vi "PCUI.vi"() -> ()   [LabVIEW 2013, in "PLTarget PC.lvclass"]
doc: "This VI is a template of the minimun components for a node UI.\nIt shows how to use the queue and the user event."
uses:
  PLTarget PC.lvclass
  <vilib>/NI/Configuration Framework/Node/NodeRef.ctl
  <vilib>/NI/Configuration Framework/Node/NISE_CEF_Node.lvclass
  <vilib>/NI/AMC/Message Queue.ctl
  <vilib>/NI/AMC/Message.ctl
  <vilib>/NI/Tools/Keyed Array/KeyedArray.ctl
  <vilib>/NI/Configuration Framework/Node/UserEventRef.ctl
  <vilib>/NI/Configuration Framework/Controls/EventCluster.ctl
  <vilib>/NI/Configuration Framework/Node/RefreshUIEvent.ctl
  <vilib>/NI/Configuration Framework/Node/CacheState.ctl
  <vilib>/NI/Configuration Framework/Node/StopEvent.ctl
  <vilib>/NI/Configuration Framework/Node/NodeChangeEvent.ctl
  <vilib>/Utility/miscctls.llb/LVPositionTypeDef.ctl
  PLTarget PC.lvclass/PLTarget PC.ctl
  Framework Configuration Classes/target configuration/PL_Target Configuration.lvclass/PL_Target Configuration.ctl
  <vilib>/NI/Configuration Framework/serializable node/NISE_CEF_serializable node.lvclass
  <vilib>/NI/Tag Bus Module Framework/root configuration/TBM configuration.lvclass
  <vilib>/NI/Configuration Framework/serializable configuration/set alias.vi
  <vilib>/NI/Configuration Framework/serializable configuration/get alias.vi
  <vilib>/NI/Configuration Framework/serializable configuration/NISE_CEF_serializable configuration.lvclass
  Framework Configuration Classes/target configuration/PL_Target Configuration.lvclass
  <vilib>/NI/DCAF UI Toolkit/Controls/DCAF UI Elements.lvlib
  <vilib>/NI/Tools/Keyed Array/Tools_KeyedArray.lvlib
  <vilib>/NI/AMC/AMC.lvlib
  <vilib>/NI/Configuration Framework/NISE_CEF_TreeControl.lvlib
panel:
  in  "Top Level Tab Control":enum32{"Configuration"}(tab)
  in  "Name":string
  in  "Includes file path":path
  in  "path to deploy on target relative to root (c:\\ or /home/lvuser/)":path
  in  "generate includes file":bool
  in  "node change":T1
  in  "stop event":T2
  in  "cache state":T3
  in  "refresh UI":T4
  in  "open fp?":bool=TRUE
  in  "user event":T5
  in  "main queue":T6
  in  "node ref":T7
  # "Target Information"
  # "Deployment Settings"
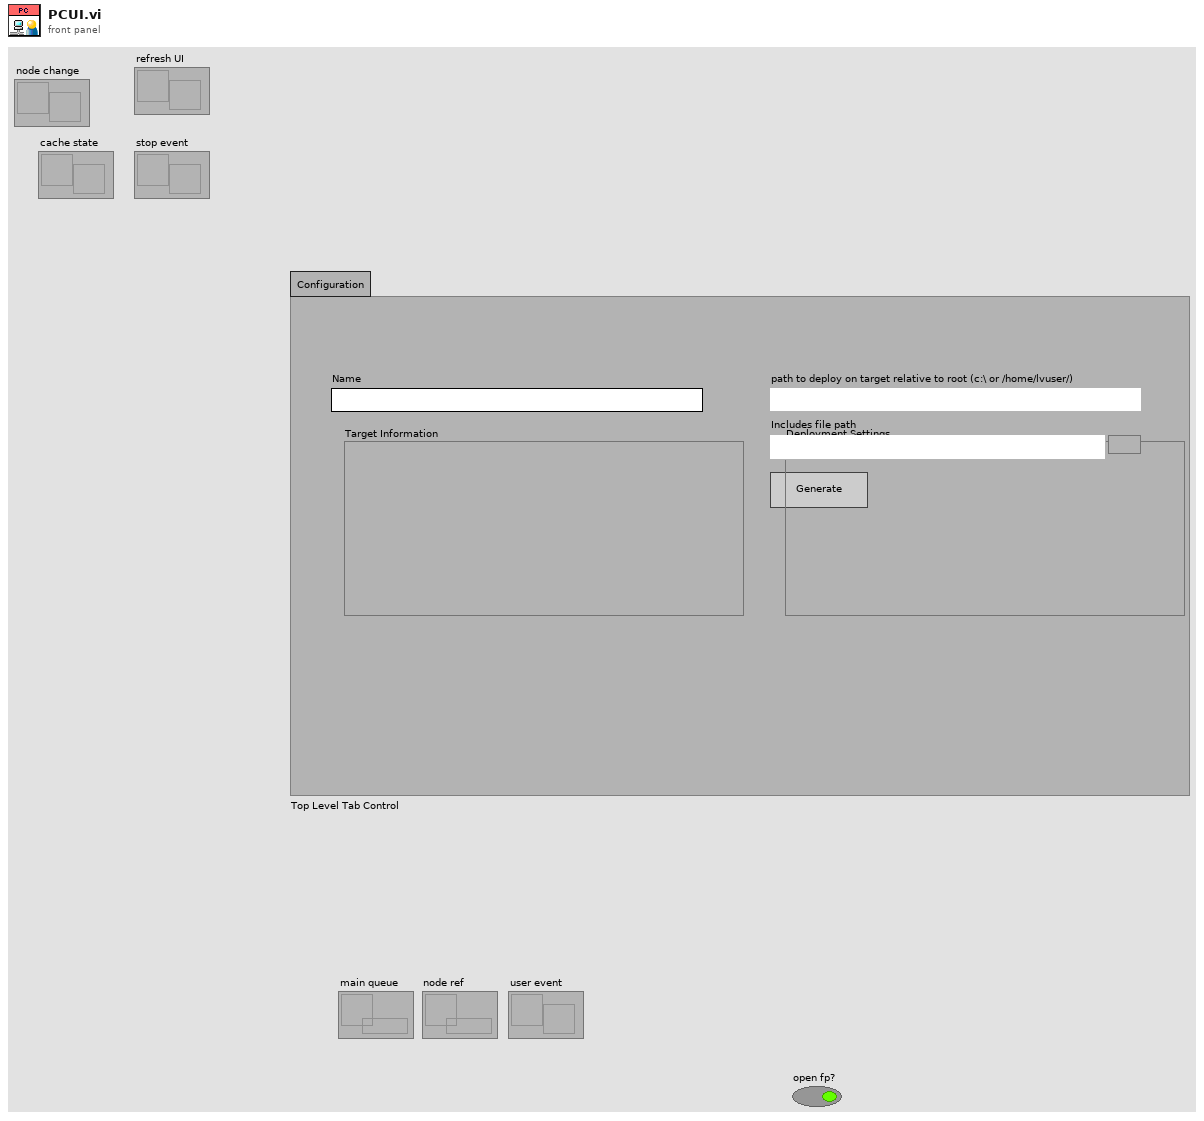
[diagram p1: front panel]
types:
  T1 = typedef "NISE_CEF_Node.lvclass/NodeChangeEvent.ctl" = refnum<user-event>
  T2 = typedef "NISE_CEF_Node.lvclass/StopEvent.ctl" = refnum<user-event>
  T3 = typedef "NISE_CEF_Node.lvclass/CacheState.ctl" = refnum<user-event>
  T4 = typedef "NISE_CEF_Node.lvclass/RefreshUIEvent.ctl" = refnum<user-event>
  T5 = typedef "NISE_CEF_Node.lvclass/UserEventRef.ctl" = refnum<user-event>
  T6 = typedef "AMC.lvlib/Message Queue.ctl" = refnum<queue>
  T7 = typedef "NISE_CEF_Node.lvclass/NodeRef.ctl" = refnum<data-value>
  T8 = typedef "LVPositionTypeDef.ctl" = cluster{"Left":i32, "Top":i32}
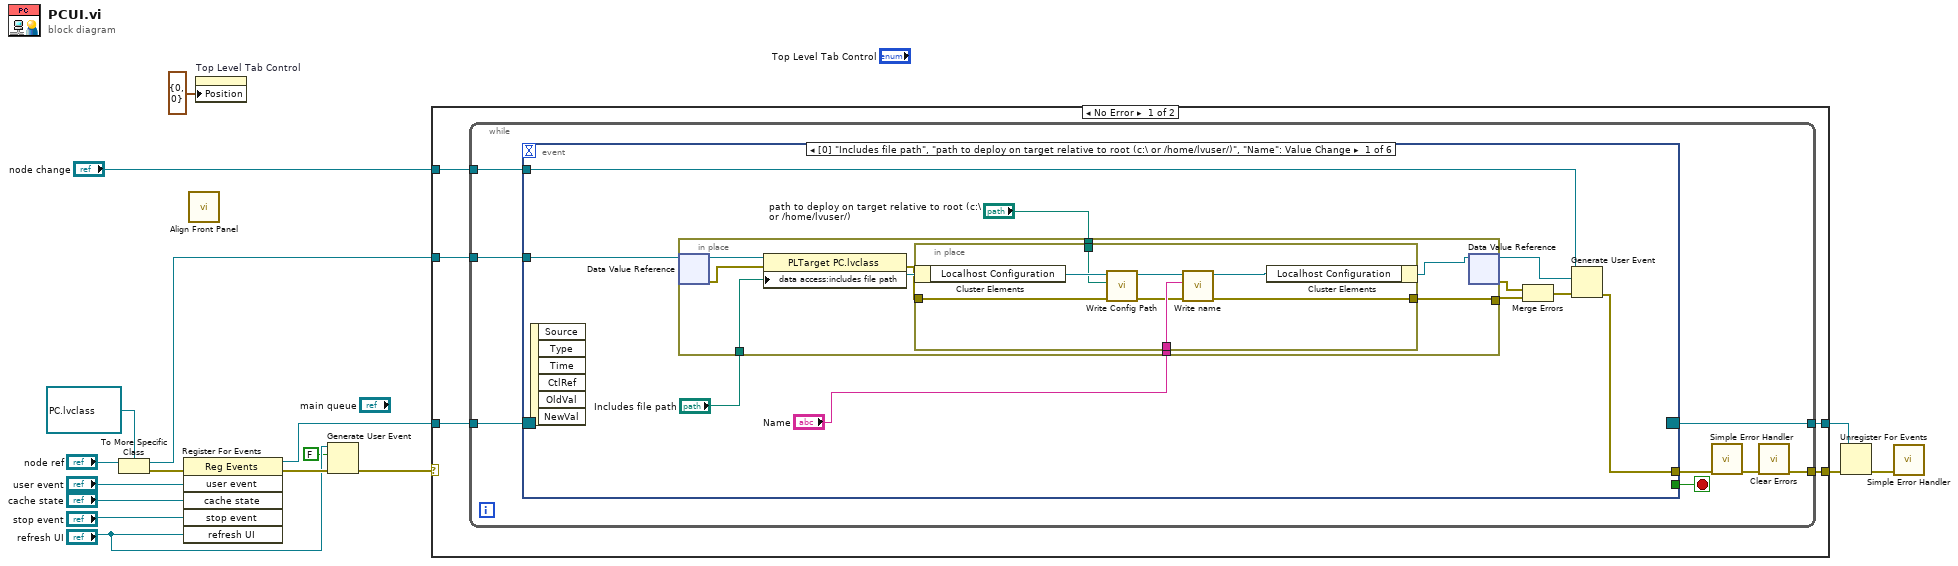
[diagram p0: block diagram]
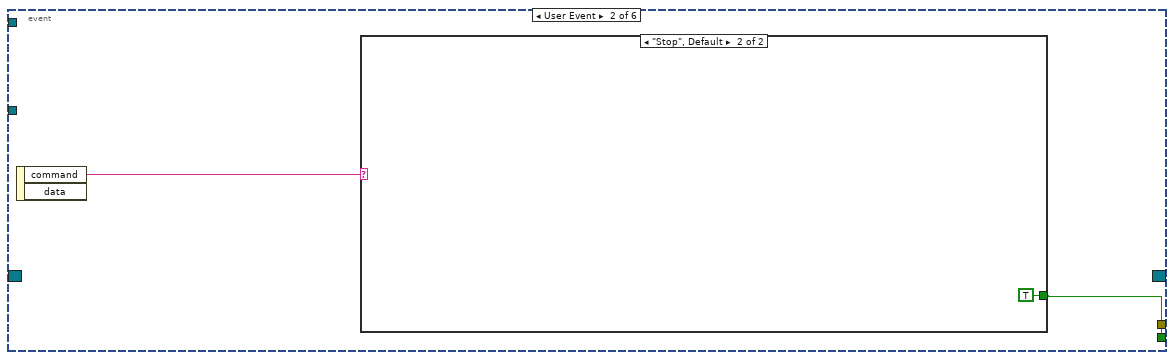
[diagram p2: hidden frame]
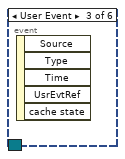
[diagram p4: hidden frame]
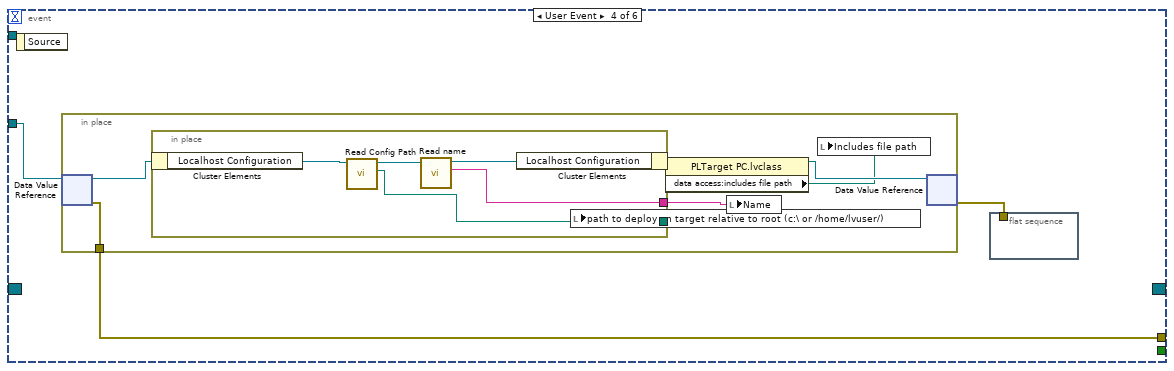
[diagram p5: hidden frame]
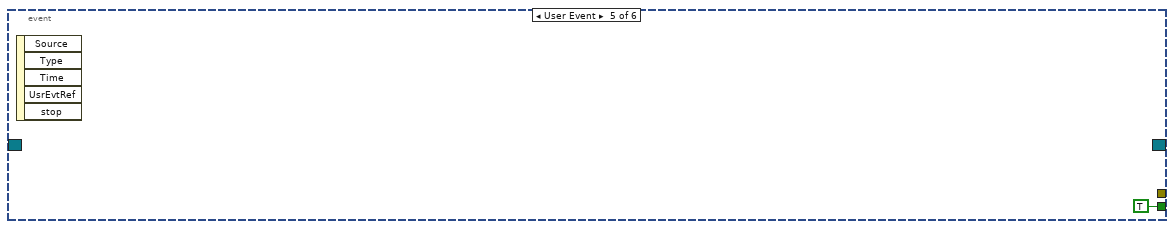
[diagram p6: hidden frame]
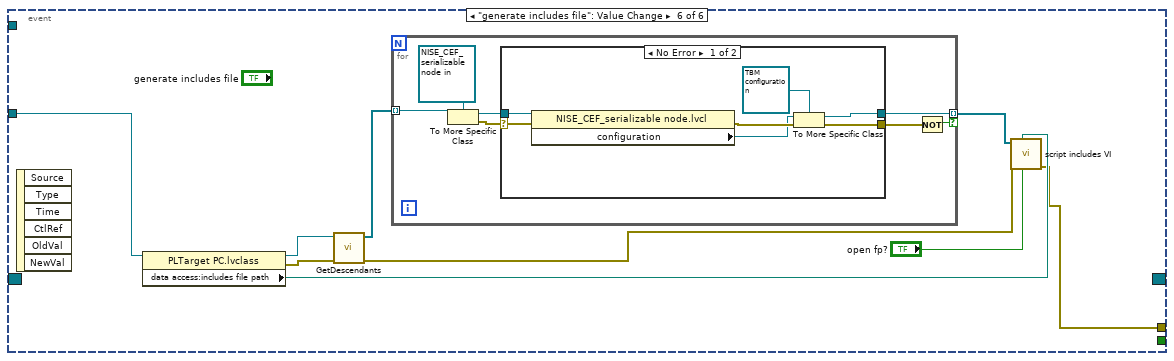
[diagram p7: hidden frame]
diagram:
  n1 = To More Specific Class(target class=refnum<data-value> refnum ("data value reference"), reference="node ref") -> (specific class reference=w4:refnum<data-value>, error out=w3:errorcluster)  [unwired: 1 in]
  n2 = register-events(error in=w3, "user event", "cache state", "stop event", "refresh UI") -> (reference out=w16:refnum<event-registration>, error out=w13:errorcluster)  [unwired: 1 in]
  n3 = call <vilib>:"Align Front Panel.vi"() -> ()  [unwired: 10 in, 2 out]
  n4 = property on="Top Level Tab Control" class="TabCtl (strict)"("Position"=T8 {"Left"=0, "Top"=0}) -> ()  [unwired: 2 in, 2 out]
  n5 = Generate User Event(user event="refresh UI", event data cluster=FALSE ("event data"), error in=w13) -> (error out=w6:errorcluster)  [unwired: 1 in, 1 out]
  n6 = case shown="No Error" w6 {
    selector: w6 -> [_ w102]
    tunnel: w4 -> [w22 _]
    tunnel: w16 -> [w21 w101]
    tunnel: [w20 w101] -> w15
    tunnel: [w19 w102] -> w14
    tunnel: "node change" -> [w18 _]
    frame No Error {
      n7 = while {
        tunnel: w22 -> [w30]
        tunnel: w21 -> [w29]
        tunnel: [w28] -> w20
        tunnel: [w24] -> w19
        tunnel: w18 -> [w23]
        stop <- w27 stop-if-true
        n8 = event shown="[0] \"Includes file path\", \"path to deploy on target relative to root (c:\\ or /home/lvuser/)\", \"Name\": Value Change" {
          selector: w29 -> [_ _ _ _ _ _]
          dyn-events: [_ _ _ _ _ _] -> w28
          timeout: _ -> [_ _ _ _ _ _]
          tunnel: w30 -> [w40 _ _ w63 _ w77]
          tunnel: [_ w59 _ _ TRUE _] -> w27
          tunnel: [w34 _ _ w62 _ w78] -> w26
          tunnel: w23 -> [w35 _ _ _ _ _]
          event "Includes file path", "path to deploy on target relative to root (c:\\ or /home/lvuser/)", "Name": Value Change {
            n9 = event-data() -> ()  [unwired: 1 in, 6 out]
            n10 = in-place {
              in-place-border: "path to deploy on target relative to root (c:\\ or /home/lvuser/)" -> [w46]
              in-place-border: "Name" -> [w45]
              in-place-border: "Includes file path" -> [w44]
              in-place-border: [w41] -> w39
              n11 = in-place-dvr #1(w40) -> (w48:refnum<class "PLTarget PC.lvclass">, w43:errorcluster)
              n12 = property class="PLTarget PC.lvclass"(reference=w48, error in=w43, "data access:includes file path"=w44) -> (reference out=w47:refnum<class "PLTarget PC.lvclass">, error out=w42:errorcluster)
              n13 = in-place {
                in-place-border: w46 -> [w54]
                in-place-border: w45 -> [w53]
                in-place-border: w42 -> [w52]
                in-place-border: [w50] -> w41
                n14 = in-place-cluster #2(w47) -> ("Localhost Configuration"=w56:refnum<class "PL_Target Configuration.lvclass">)
                n15 = call "Write Config Path.vi"("error in"=w52, "Config Path"=w54, "PL_Local Target Configuration in"=w56) -> ("error out"=w51:errorcluster, "PL_Local Target Configuration out"=w57:refnum<class "PL_Target Configuration.lvclass">)  [unwired: 7 in]
                n16 = call "Write name.vi"("error in"=w51, "name"=w53, "PL_Local Target Configuration in"=w57) -> ("error out"=w50:errorcluster, "PL_Local Target Configuration out"=w55:refnum<class "PL_Target Configuration.lvclass">)  [unwired: 7 in]
                n17 = in-place-cluster #2("Localhost Configuration"=w55) -> (w49:refnum<class "PLTarget PC.lvclass">)
              }
              n18 = in-place-dvr #1(w49) -> (w36:refnum<data-value>, w38:errorcluster)
            }
            n19 = Merge Errors(w38, w39) -> (w37:errorcluster)
            n20 = Generate User Event(user event=w35, event data cluster=w36, error in=w37) -> (error out=w34:errorcluster)  [unwired: 1 in, 1 out]
          }
          event User Event {
            n21 = event-data() -> ("command"=w58:string)  [unwired: 1 in, 1 out]
            n22 = case shown="\"Stop\", Default" w58 {
              tunnel: [_ TRUE] -> w59
              frame "Refresh", "Save" {
              }
              frame "Stop", Default {
              }
            }
          }
          event User Event {
            n23 = event-data() -> ()  [unwired: 1 in, 5 out]
          }
          event User Event {
            n24 = event-data() -> ()  [unwired: 1 in, 1 out]
            n25 = in-place {
              in-place-border: [w67] -> w62
              n26 = in-place-dvr #3(w63) -> (w68:refnum<class "PLTarget PC.lvclass">, w67:errorcluster)
              n27 = in-place {
                in-place-border: [w75] -> w70
                in-place-border: [w74] -> w69
                n28 = in-place-cluster #4(w68) -> ("Localhost Configuration"=w72:refnum<class "PL_Target Configuration.lvclass">)
                n29 = call "Read Config Path.vi"("PL_Local Target Configuration in"=w72) -> ("Config Path"=w75:path, "PL_Local Target Configuration out"=w73:refnum<class "PL_Target Configuration.lvclass">)  [unwired: 8 in, 1 out]
                n30 = call "Read name.vi"("PL_Local Target Configuration in"=w73) -> ("name"=w74:string, "PL_Local Target Configuration out"=w71:refnum<class "PL_Target Configuration.lvclass">)  [unwired: 8 in, 1 out]
                n31 = in-place-cluster #4("Localhost Configuration"=w71) -> (w66:refnum<class "PLTarget PC.lvclass">)
              }
              n32 = local write "path to deploy on target relative to root (c:\\ or /home/lvuser/)"(w70) -> ()
              n33 = property class="PLTarget PC.lvclass"(reference=w66) -> (reference out=w65:refnum<class "PLTarget PC.lvclass">, "data access:includes file path"=w64:path)  [unwired: 1 in, 1 out]
              n34 = local write "Name"(w69) -> ()
              n35 = local write "Includes file path"(w64) -> ()
              n36 = in-place-dvr #3(w65) -> (w61:errorcluster)  [unwired: 1 out]
            }
            n37 = flat-sequence {
              tunnel: w61 -> [_]
              frame #0 {
              }
            }
          }
          event User Event {
            n38 = event-data() -> ()  [unwired: 1 in, 5 out]
          }
          event "generate includes file": Value Change {
            n39 = event-data() -> ()  [unwired: 1 in, 6 out]
            n40 = property class="PLTarget PC.lvclass"(reference=w77) -> (reference out=w83:refnum<data-value>, error out=w82:errorcluster, "data access:includes file path"=w81:path)  [unwired: 1 in]
            n41 = call <vilib>:"GetDescendants.vi"("error in"=w82, "node in"=w83) -> ("error out"=w79:errorcluster, "descendants"=w84:refnum<data-value>[])  [unwired: 8 in]
            n42 = for {
              tunnel: w84 -> [w92] mode=indexing
              tunnel: [w88] -> w85 mode=indexing if=w86
              n43 = To More Specific Class(target class=refnum<data-value> refnum, reference=w92) -> (specific class reference=w89:refnum<data-value>, error out=w90:errorcluster)  [unwired: 1 in]
              n44 = case shown="No Error" w90 {
                selector: w90 -> [w98 w100]
                tunnel: w89 -> [w99 _]
                tunnel: [w93 _] -> w88
                tunnel: [w96 w100] -> w87
                frame No Error {
                  n45 = property class="NISE_CEF_serializable node.lvcl"(reference=w99, error in=w98) -> (error out=w97:errorcluster, "configuration"=w95:refnum<class "NISE_CEF_serializable configuration.lvclass">)  [unwired: 1 out]
                  n46 = To More Specific Class(target class=refnum<class "TBM configuration.lvclass"> refnum ("configuration"), reference=w95, error in=w97) -> (specific class reference=w93:refnum<class "TBM configuration.lvclass">, error out=w96:errorcluster)
                }
                frame Error {
                }
              }
              n47 = Not(x=w87) -> (.not. x?=w86:bool)
            }
            n48 = call "script includes VI.vi"("open fp?"="open fp?", "vi path (blank=new)"=w81, "error in"=w79, "cfg objects"=w85) -> ("error out"=w78:errorcluster)  [unwired: 7 in]
          }
        }
        n49 = call <vilib>:"Simple Error Handler.vi"("error in (no error)"=w26) -> ("error out"=w25:errorcluster)  [unwired: 4 in, 4 out]
        n50 = call <vilib>:"Clear Errors.vi"("error in (no error)"=w25) -> ("error out"=w24:errorcluster)  [unwired: 6 in]
      }
    }
    frame Error {
    }
  }
  n51 = Unregister For Events(event registration refnum=w15, error in=w14) -> (error out=w5:errorcluster)
  n52 = call <vilib>:"Simple Error Handler.vi"("error in (no error)"=w5) -> ()  [unwired: 4 in, 5 out]
